vi "Calculate Distance Loop.vi"(7 "Position And Thickness":refnum<notifier>, 8 "error in (no error)":errorcluster caption="错误输入（无错误）", 9 "DSP Signal":refnum<notifier>, 10 "CDL":refnum<queue>, 11 "Director":refnum<queue>) -> (0 "error out":errorcluster caption="错误输出")   [LabVIEW 2015, in "Boimetry Processing.lvlib"]
doc: "该消息循环负责处理硬件数据采集的相关消息。"
uses:
  Boimetry Processing.lvlib
  support/Message Queue/Message Cluster.ctl
  Controls/Calculating Distance State.ctl
  Controls/Biometry Configuration.ctl
  support/Message Queue/Enqueue Message (Single).vi
  <vilib>/Utility/error.llb/Error Cluster From Error Code.vi
  <vilib>/ErrorRing/Error Ring.xnode
  support/Message Queue/Message Queue.lvlib
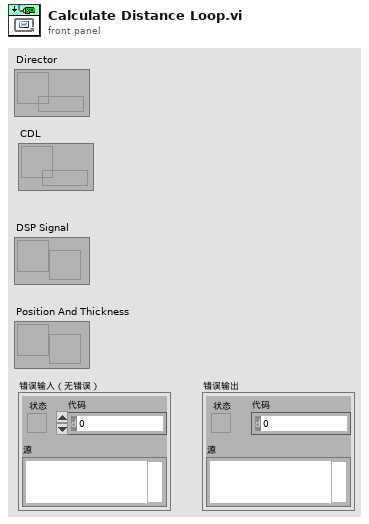
[diagram p1: front panel]
types:
  T1 = typedef "Boimetry Processing.lvlib/Biometry Configuration.ctl" = cluster{"Interference Width":i32, "Interference Threshold":dbl, "Cornea Len Division":i32, "Correction Data 1st Path":string, "1st_Start_Position":dbl, "Correction Data 2nd Path":string, "2nd_Start_Position":dbl, "Index Corneal":dbl, "Index Water":dbl, "Index Len":dbl, "Working Position":cluster{"FirstStart":i32, "FirstEnd":i32, "SecondStart":i32, "SecondEnd":i32}}
  T2 = typedef "Boimetry Processing.lvlib/Calculating Distance State.ctl" = enum16{"Idle", "Calculating"}
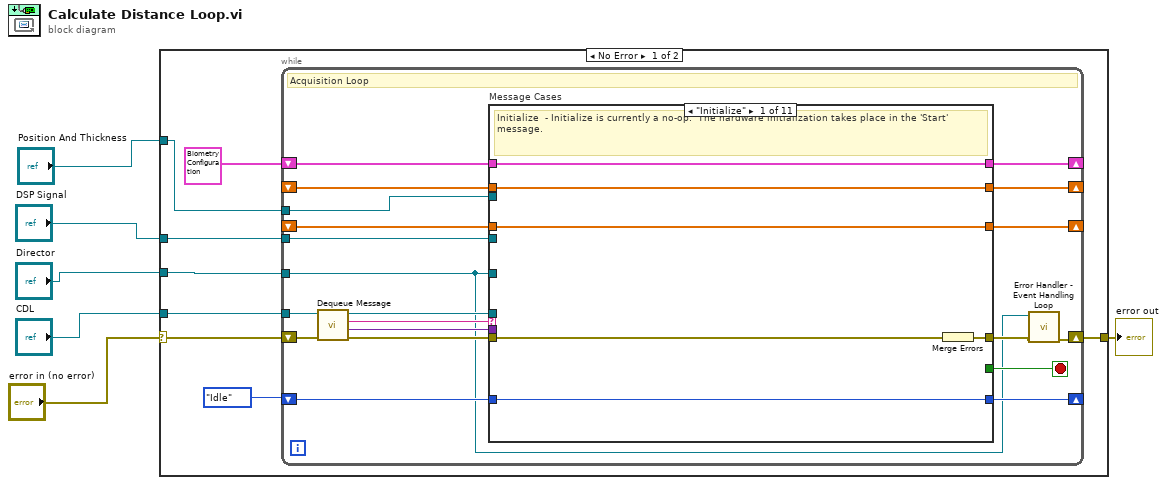
[diagram p0: block diagram]
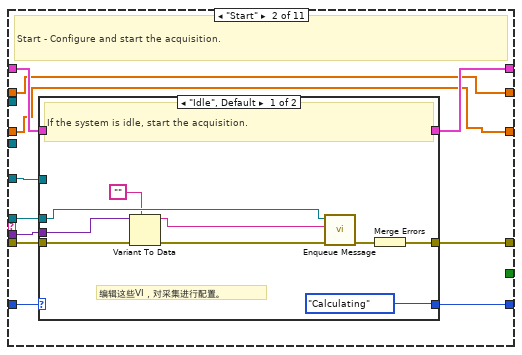
[diagram p2: hidden frame]
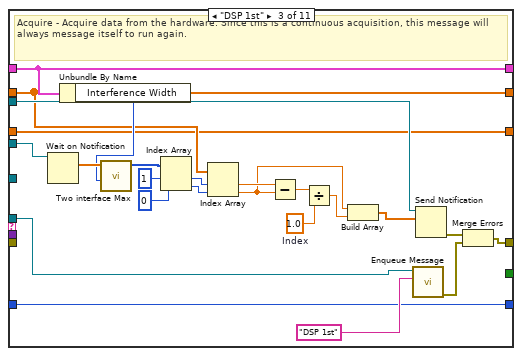
[diagram p4: hidden frame]
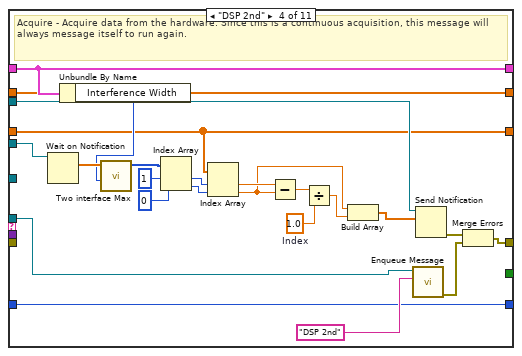
[diagram p5: hidden frame]
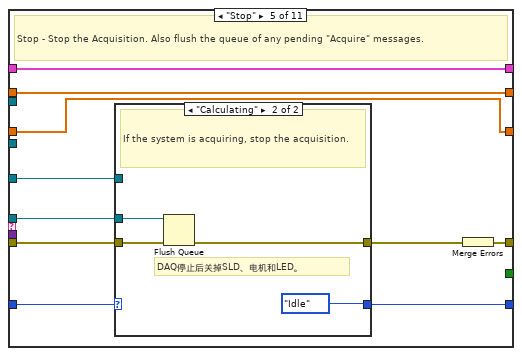
[diagram p6: hidden frame]
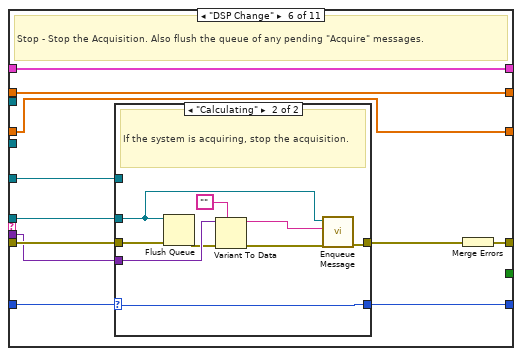
[diagram p8: hidden frame]
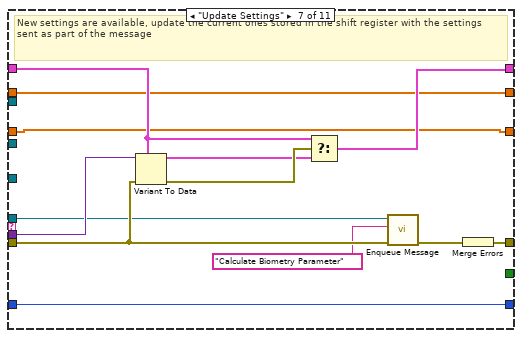
[diagram p10: hidden frame]
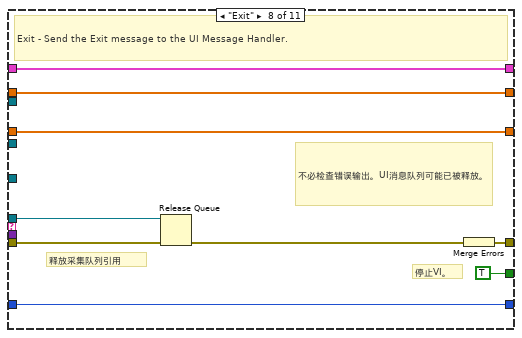
[diagram p11: hidden frame]
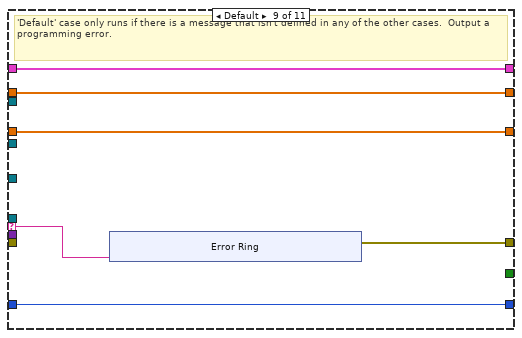
[diagram p12: hidden frame]
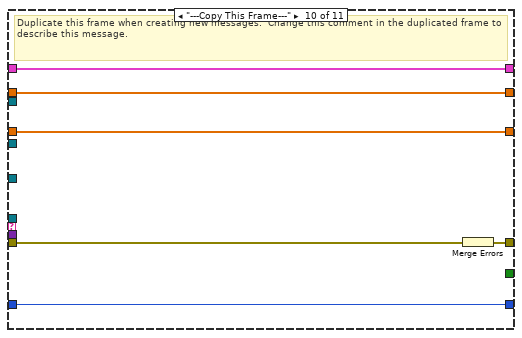
[diagram p13: hidden frame]
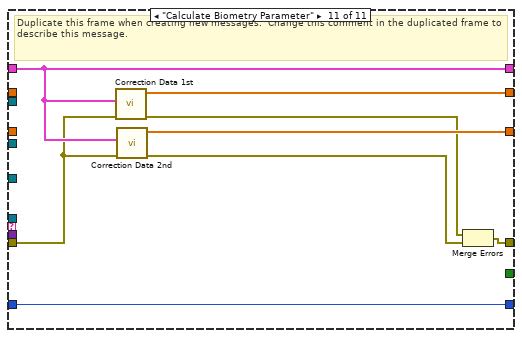
[diagram p14: hidden frame]
diagram:
  n1 = case shown="No Error" "error in (no error)" {
    selector: "error in (no error)" -> [w13 w200]
    tunnel: [w14 w200] -> w6
    tunnel: "DSP Signal" -> [w12 _]
    tunnel: "CDL" -> [w11 _]
    tunnel: "Director" -> [w10 _]
    tunnel: "Position And Thickness" -> [w9 _]
    frame No Error {
      n2 = while {
        tunnel: w11 -> [w26]
        shift-right: [w33] -> _
        shift-left: T1 {"Interference Width"=0, "Interference Threshold"=0.0, "Cornea Len Division"=0, "Correction Data 1st Path"="", "1st_Start_Position"=0.0, "Correction Data 2nd Path"="", "2nd_Start_Position"=0.0, "Index Corneal"=0.0, "Index Water"=0.0, "Index Len"=0.0, "Working Position"={"FirstStart"=0, "FirstEnd"=0, "SecondStart"=0, "SecondEnd"=0}} ("Biometry Configuration") -> [w34]
        shift-right: [w23] -> w14
        shift-left: w13 -> [w31]
        tunnel: w10 -> [w21]
        shift-right: [w24] -> _
        shift-left: Calculating_Distance_State."Idle" ("记录状态") -> [w25]
        tunnel: w12 -> [w20]
        tunnel: w9 -> [w19]
        shift-right: [w18] -> _
        shift-left: _ -> [w16]
        shift-right: [w17] -> _
        shift-left: _ -> [w15]
        stop <- w32 stop-if-true
        # "Acquisition Loop"
        n3 = call "Dequeue Message.vi"("error in (no error)"=w31, "消息队列"=w26) -> ("error out"=w30:cluster{"状态":bool, "代码":i32, "源":string}, "消息数据"=w28:variant, "消息"=w29:string, "消息队列副本"=w27:refnum<queue>)  [unwired: 6 in]
        n4 = case "Message Cases" shown="\"Initialize\"" w29 {
          selector: w29 -> [_ _ _ _ _ _ _ _ w177 _ _]
          tunnel: w27 -> [_ w48 w86 w110 w119 w136 w154 w169 _ _ _]
          tunnel: w30 -> [w38 w49 _ _ w121 w138 w156 w166 _ w191 w196]
          tunnel: [w40 w51 w88 w112 w122 w139 w163 w171 w176 w189 w199] -> w22
          tunnel: w34 -> [w37 w50 w79 w103 w120 w137 w159 w167 w178 w190 w197]
          tunnel: [w37 w47 w79 w103 w120 w137 w158 w167 w178 w190 w197] -> w33
          tunnel: [_ _ _ _ _ _ _ TRUE _ _ _] -> w32
          tunnel: w28 -> [_ w43 _ _ _ w131 w162 _ _ _ _]
          tunnel: w21 -> [_ w44 _ _ w118 w135 _ _ _ _ _]
          tunnel: w25 -> [w39 w46 w84 w108 w117 w134 w157 w168 w175 w188 w198]
          tunnel: [w39 w45 w84 w108 w116 w133 w157 w168 w175 w188 w198] -> w24
          tunnel: w20 -> [_ _ w82 w106 _ _ _ _ _ _ _]
          tunnel: w19 -> [_ _ w81 w105 _ _ _ _ _ _ _]
          tunnel: [w36 w42 w66 w90 w114 w130 w152 w165 w174 w187 w195] -> w18
          tunnel: [w35 w41 w65 w89 w113 w129 w151 w164 w173 w186 w194] -> w17
          tunnel: w16 -> [w36 w42 w66 w90 w114 w130 w152 w165 w174 w187 _]
          tunnel: w15 -> [w35 w41 w65 w89 w113 w129 w151 w164 w173 w186 _]
          frame "Initialize" {
            # "Initialize  - Initialize is currently a no-op.  The hardware initialization takes place in the 'Start' message."
            n5 = Merge Errors(w38) -> (w40:errorcluster)
          }
          frame "Start" {
            # "Start - Configure and start the acquisition."
            n6 = case shown="\"Idle\", Default" w46 {
              selector: w46 -> [_ w62]
              tunnel: [w61 w64] -> w51
              tunnel: w50 -> [w58 w63]
              tunnel: w49 -> [w57 w64]
              tunnel: w48 -> [w59 _]
              tunnel: [w58 w63] -> w47
              tunnel: [Calculating_Distance_State."Calculating" ("记录状态") w62] -> w45
              tunnel: w44 -> [_ _]
              tunnel: w43 -> [w55 _]
              frame "Idle", Default {
                # "编辑这些VI，对采集进行配置。"
                # "If the system is idle, start the acquisition."
                n7 = Variant To Data(error in=w57, type="", Variant=w55) -> (data=w53:string, error out=w56:errorcluster)
                n8 = call-poly "Enqueue Message.vi"("error in (no error)"=w56, "消息"=w53, "消息队列"=w59) -> ("error out"=w60:cluster{"状态":bool, "代码":i32, "源":string})  [unwired: 7 in, 1 out]
                n9 = Merge Errors(w60) -> (w61:errorcluster)
              }
              frame "Calculating" {
                # "The system is already acquiring. Ignore the \"Start\" message."
              }
            }
          }
          frame "DSP 1st" {
            w70 = 1.0  # Index
            # "Acquire - Acquire data from the hardware. Since this is a continuous acquisition, this message will always message itself to run again."
            n10 = Wait on Notification(notifier=w82) -> (notification=w80:dbl[])  [unwired: 3 in, 3 out]
            n11 = Unbundle By Name(w79) -> ("Interference Width"=w78:i32)
            n12 = call "Two interface Max.vi"("Width"=w78, "S"=w80) -> ("INDEX"=w77:i32[])  [unwired: 8 in, 1 out]
            n13 = Index Array(array=w77, index #1=1 ("索引"), index #2=0 ("索引")) -> (element #1=w74:i32, element #2=w73:i32)
            n14 = Index Array(array=w66, index #1=w74, index #2=w73) -> (element #1=w72:dbl, element #2=w69:dbl)
            n15 = Subtract(x=w72, y=w69) -> (x-y=w71:dbl)
            n16 = Divide(x=w71, y=w70) -> (x/y=w68:dbl)
            n17 = Build Array(w69, w68) -> (w67:dbl[])
            n18 = call-poly "Enqueue Message.vi"("消息"="DSP 1st" ("Message"), "消息队列"=w86) -> ("error out"=w87:cluster{"状态":bool, "代码":i32, "源":string})  [unwired: 8 in, 1 out]
            n19 = Send Notification(notification=w67, notifier=w81) -> (error out=w83:errorcluster)  [unwired: 1 in, 1 out]
            n20 = Merge Errors(w83, w87) -> (w88:errorcluster)
          }
          frame "DSP 2nd" {
            w94 = 1.0  # Index
            # "Acquire - Acquire data from the hardware. Since this is a continuous acquisition, this message will always message itself to run again."
            n21 = Wait on Notification(notifier=w106) -> (notification=w104:dbl[])  [unwired: 3 in, 3 out]
            n22 = Unbundle By Name(w103) -> ("Interference Width"=w102:i32)
            n23 = call "Two interface Max.vi"("Width"=w102, "S"=w104) -> ("INDEX"=w101:i32[])  [unwired: 8 in, 1 out]
            n24 = Index Array(array=w101, index #1=1 ("索引"), index #2=0 ("索引")) -> (element #1=w98:i32, element #2=w97:i32)
            n25 = Index Array(array=w89, index #1=w98, index #2=w97) -> (element #1=w96:dbl, element #2=w93:dbl)
            n26 = Subtract(x=w96, y=w93) -> (x-y=w95:dbl)
            n27 = Divide(x=w95, y=w94) -> (x/y=w92:dbl)
            n28 = Build Array(w93, w92) -> (w91:dbl[])
            n29 = call-poly "Enqueue Message.vi"("消息"="DSP 2nd" ("Message"), "消息队列"=w110) -> ("error out"=w111:cluster{"状态":bool, "代码":i32, "源":string})  [unwired: 8 in, 1 out]
            n30 = Send Notification(notification=w91, notifier=w105) -> (error out=w107:errorcluster)  [unwired: 1 in, 1 out]
            n31 = Merge Errors(w107, w111) -> (w112:errorcluster)
          }
          frame "Stop" {
            # "Stop - Stop the Acquisition. Also flush the queue of any pending \"Acquire\" messages."
            n32 = case shown="\"Calculating\"" w117 {
              selector: w117 -> [w124 _]
              tunnel: w121 -> [w123 w128]
              tunnel: w119 -> [_ w127]
              tunnel: w118 -> [_ _]
              tunnel: [w124 Calculating_Distance_State."Idle" ("记录状态")] -> w116
              tunnel: [w123 w126] -> w115
              frame "Idle", Default {
                # "The system is already idle. Ignore the \"Stop\" message."
              }
              frame "Calculating" {
                # "DAQ停止后关掉SLD、电机和LED。"
                # "If the system is acquiring, stop the acquisition."
                n33 = Flush Queue(queue=w127, error in (no error)=w128) -> (error out=w126:errorcluster)  [unwired: 2 out]
              }
            }
            n34 = Merge Errors(w115) -> (w122:errorcluster)
          }
          frame "DSP Change" {
            # "Stop - Stop the Acquisition. Also flush the queue of any pending \"Acquire\" messages."
            n35 = case shown="\"Calculating\"" w134 {
              selector: w134 -> [w141 w149]
              tunnel: w138 -> [w140 w150]
              tunnel: w136 -> [_ w147]
              tunnel: w135 -> [_ _]
              tunnel: [w141 w149] -> w133
              tunnel: [w140 w148] -> w132
              tunnel: w131 -> [_ w146]
              frame "Idle", Default {
                # "The system is already idle. Ignore the \"Stop\" message."
              }
              frame "Calculating" {
                # "If the system is acquiring, stop the acquisition."
                n36 = Flush Queue(queue=w147, error in (no error)=w150) -> (error out=w144:errorcluster)  [unwired: 2 out]
                n37 = Variant To Data(error in=w144, type="", Variant=w146) -> (data=w142:string, error out=w143:errorcluster)
                n38 = call-poly "Enqueue Message.vi"("error in (no error)"=w143, "消息"=w142, "消息队列"=w147) -> ("error out"=w148:cluster{"状态":bool, "代码":i32, "源":string})  [unwired: 7 in, 1 out]
              }
            }
            n39 = Merge Errors(w132) -> (w139:errorcluster)
          }
          frame "Update Settings" {
            # "New settings are available, update the current ones stored in the shift register with the settings sent as part of the message"
            n40 = Variant To Data(error in=w156, type=w159, Variant=w162) -> (data=w160:T1, error out=w161:errorcluster)
            n41 = Select(t=w159, s=w161, f=w160) -> (s? t:f=w158:T1)
            n42 = call-poly "Enqueue Message.vi"("error in (no error)"=w156, "消息"="Calculate Biometry Parameter", "消息队列"=w154) -> ("error out"=w155:cluster{"状态":bool, "代码":i32, "源":string})  [unwired: 7 in, 1 out]
            n43 = Merge Errors(w155) -> (w163:errorcluster)
          }
          frame "Exit" {
            # "不必检查错误输出。UI消息队列可能已被释放。"
            # "释放采集队列引用"
            # "停止VI。"
            # "Exit - Send the Exit message to the UI Message Handler."
            n44 = Release Queue(queue=w169, error in (no error)=w166) -> (error out=w170:errorcluster)  [unwired: 1 in, 2 out]
            n45 = Merge Errors(w170) -> (w171:errorcluster)
          }
          frame Default {
            # "'Default' case only runs if there is a message that isn't defined in any of the other cases.  Output a programming error."
            n46 = xnode "Error Ring"("parameter 0"=w177) -> ("error out"=w176:errorcluster)
          }
          frame "---Copy This Frame---" {
            # "Duplicate this frame when creating new messages.  Change this comment in the duplicated frame to describe this message."
            n47 = Merge Errors(w191) -> (w189:errorcluster)
          }
          frame "Calculate Biometry Parameter" {
            # "Duplicate this frame when creating new messages.  Change this comment in the duplicated frame to describe this message."
            n48 = call "Correction Data 1st.vi"("错误输入"=w196, "Biometry Configuration"=w197) -> ("错误输出"=w193:errorcluster, "Output Correction Data"=w195:dbl[])  [unwired: 8 in]
            n49 = call "Correction Data 2nd.vi"("错误输入"=w196, "Biometry Configuration"=w197) -> ("错误输出"=w192:errorcluster, "Output Correction Data"=w194:dbl[])  [unwired: 8 in]
            n50 = Merge Errors(w193, w192) -> (w199:errorcluster)
          }
        }
        n51 = call "Error Handler - Event Handling Loop.vi"("error in (no error)"=w22, "消息队列"=w21) -> ("错误输入副本"=w23:cluster{"状态":bool, "代码":i32, "源":string})  [unwired: 8 in, 1 out]
      }
    }
    frame Error {
    }
  }
  "error out" <- w6
